vi "Actor Core.vi"(8 "error in":errorcluster, 11 "Sample in":refnum<class "Sample.lvclass">) -> (0 "error out":errorcluster, 3 "Actor out":refnum<class "Actor.lvclass">)   [LabVIEW 2022 SP3, in "Sample.lvlib" / "Sample.lvclass"]
doc: "(<B>Filename</B>: Actor Framework.lvlib:Actor.lvclass:Actor Core.vi)\n\nReceives messages to the actor, reacts to them, and initiates any error handling that may shut the actor down.\n\nDescendant classes may override this VI to append parallel tasks for the actor to complete while it handles messages. Overrides use the Call Parent Class Method node."
uses:
  Sample.lvclass
  Sample.lvclass/Sample.ctl
  <vilib>/MGI/Monitored Actor/Monitored Actor/Monitored Actor/Monitored Actor.lvclass
  <vilib>/ActorFramework/Actor/Actor.lvclass
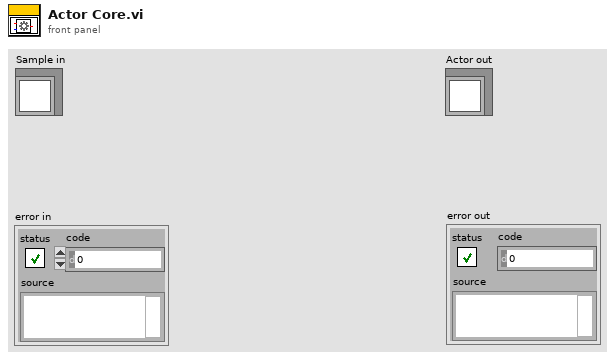
[diagram p1: front panel]
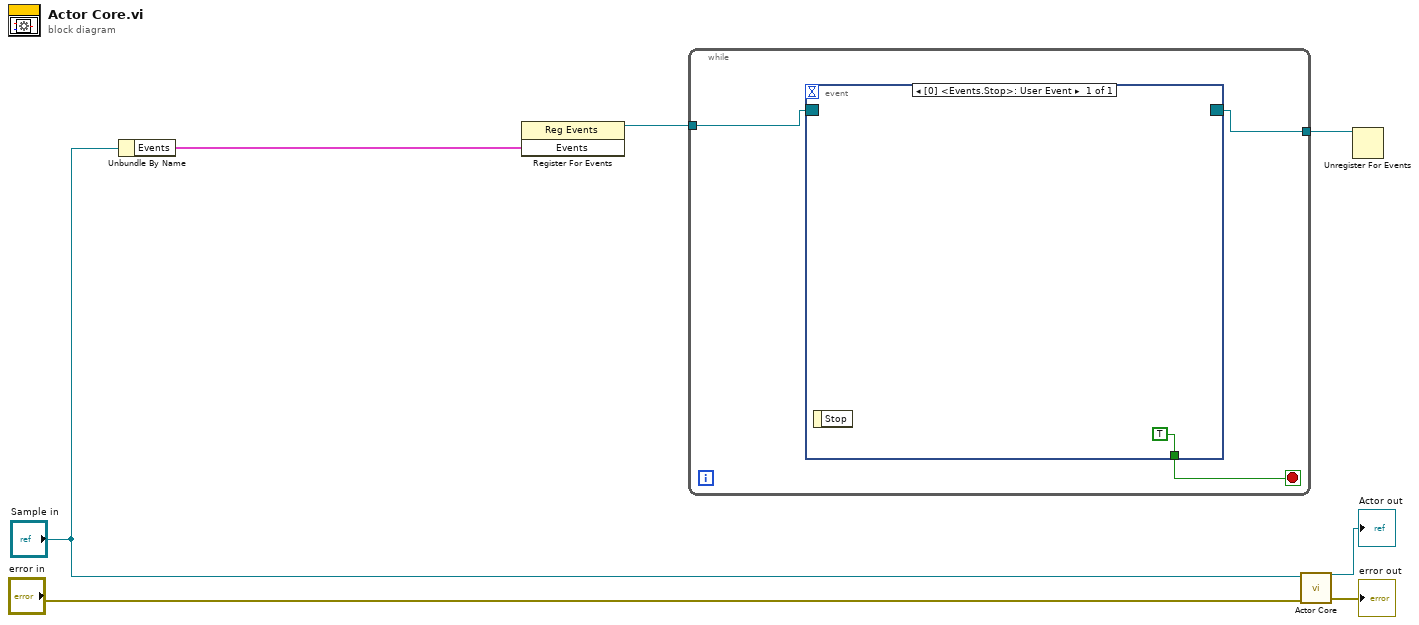
[diagram p0: block diagram]
diagram:
  n1 = Unbundle By Name("Sample in") -> ("Events"=w3:cluster{"Stop":refnum<user-event>})
  n2 = register-events(w3) -> (reference out=w2:refnum<event-registration>)  [unwired: 2 in, 1 out]
  n3 = while {
    tunnel: w2 -> [w10]
    tunnel: [w9] -> w1
    stop <- w8 stop-if-true
    n4 = event shown="[0] <Events.Stop>: User Event" {
      selector: w10 -> [_]
      dyn-events: [_] -> w9
      timeout: _ -> [_]
      tunnel: [TRUE] -> w8
      event User Event {
        n5 = event-data() -> ()  [unwired: 1 in, 1 out]
      }
    }
  }
  n6 = call-parent "Actor Core.vi"("error in"="error in", "Actor in"="Sample in") -> ("error out"=→"error out":errorcluster, "Actor out"=→"Actor out":refnum<class "Actor.lvclass">)  [unwired: 8 in]
  n7 = Unregister For Events(event registration refnum=w1) -> ()  [unwired: 1 in, 1 out]
